vi "PCO_Grab_Save.vi"(7 "# of frames":u16, 8 "entrée d'erreur (pas d'erreur)":errorcluster, 9 "Message Data":variant, 10 "notifier out":refnum<notifier>, 11 "Camera en entrée":refnum<class "Camera.lvclass">) -> (0 "sortie d'erreur":errorcluster, 1 "meta_data_list":T1(array[cluster]), 2 "Raw data (U16)":u16[][][](array[numeric]), 3 "Camera en sortie":refnum<class "Camera.lvclass">)   [LabVIEW 2026]
uses:
  pco.labview/camera/Camera.lvclass
  Controls/PCO_Config.ctl
panel:
  out "recorded_image_count":u32
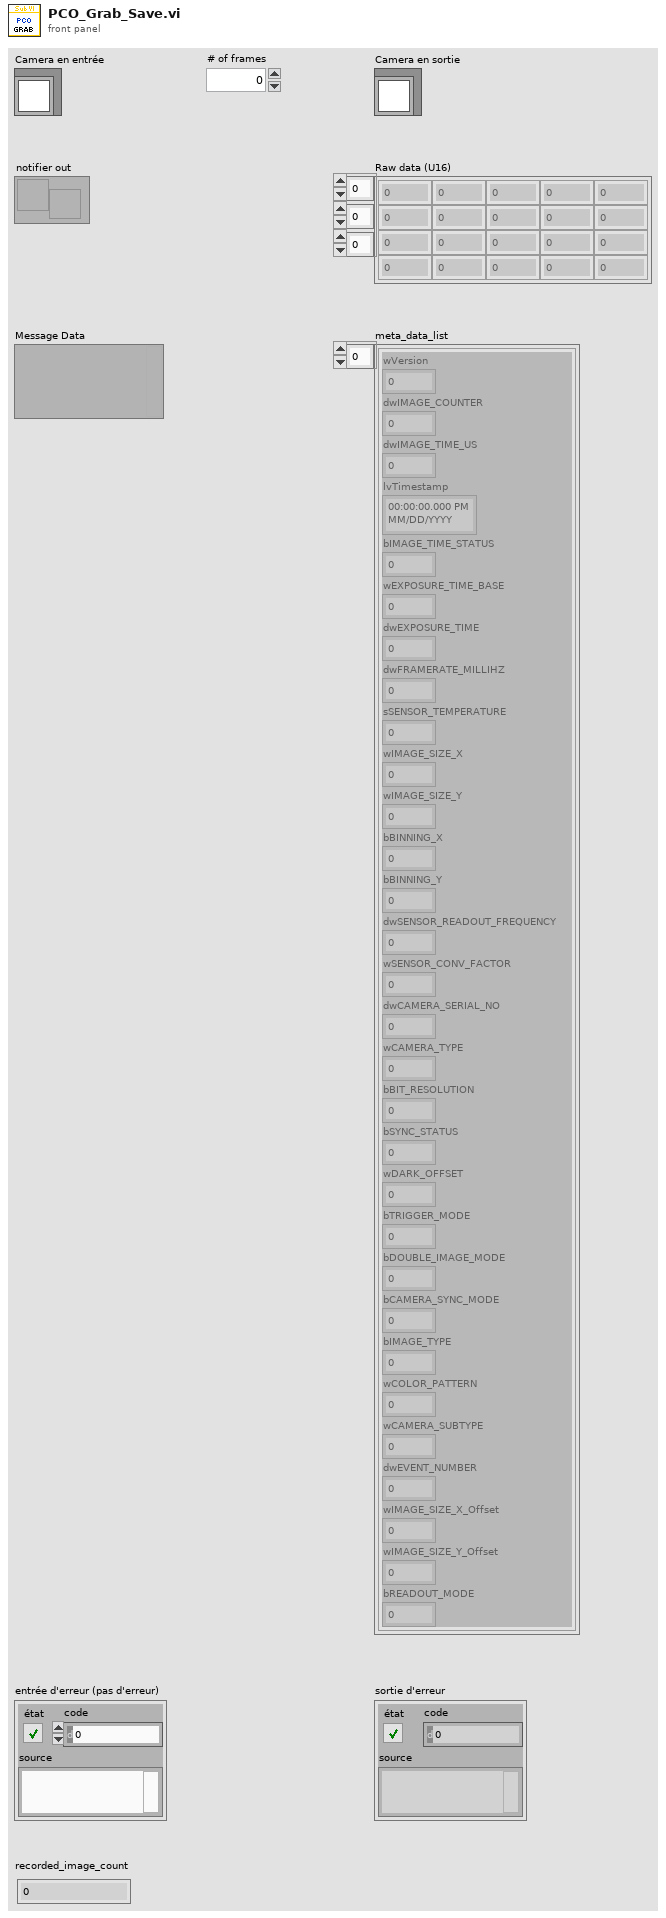
[diagram p1: front panel]
types:
  T1 = cluster{"wVersion":u16, "dwIMAGE_COUNTER":u32, "dwIMAGE_TIME_US":u32, "lvTimestamp":timestamp, "bIMAGE_TIME_STATUS":u8, "wEXPOSURE_TIME_BASE":u16, "dwEXPOSURE_TIME":u32, "dwFRAMERATE_MILLIHZ":u32, "sSENSOR_TEMPERATURE":i16, "wIMAGE_SIZE_X":u16, "wIMAGE_SIZE_Y":u16, "bBINNING_X":u8, "bBINNING_Y":u8, "dwSENSOR_READOUT_FREQUENCY":u32, "wSENSOR_CONV_FACTOR":u16, "dwCAMERA_SERIAL_NO":u32, "wCAMERA_TYPE":u16, "bBIT_RESOLUTION":u8, "bSYNC_STATUS":u8, "wDARK_OFFSET":u16, "bTRIGGER_MODE":u8, "bDOUBLE_IMAGE_MODE":u8, "bCAMERA_SYNC_MODE":u8, "bIMAGE_TYPE":u8, "wCOLOR_PATTERN":u16, "wCAMERA_SUBTYPE":u16, "dwEVENT_NUMBER":u32, "wIMAGE_SIZE_X_Offset":u16, "wIMAGE_SIZE_Y_Offset":u16, "bREADOUT_MODE":u8}[]
  T2 = enum16{"sequence", "sequence non blocking", "ring buffer", "fifo", "tif", "multitif", "pcoraw", "b16", "dicom", "multidicom", "camram_ring", "camram_segment"}
  T3 = enum16{"Undefined", "Mono8", "Mono16", "BGRA8", "RGBA8", "BGRA16", "RGBA16", "CompressedMono8"}
  T4 = typedef "PCO_Config.ctl" = cluster{"Exposure time (s)":dbl, "TriggerMode":u16, "ROI X0":u16, "ROI Y0":u16, "ROI X1":u16, "ROI Y1":u16, "Binning":u8}
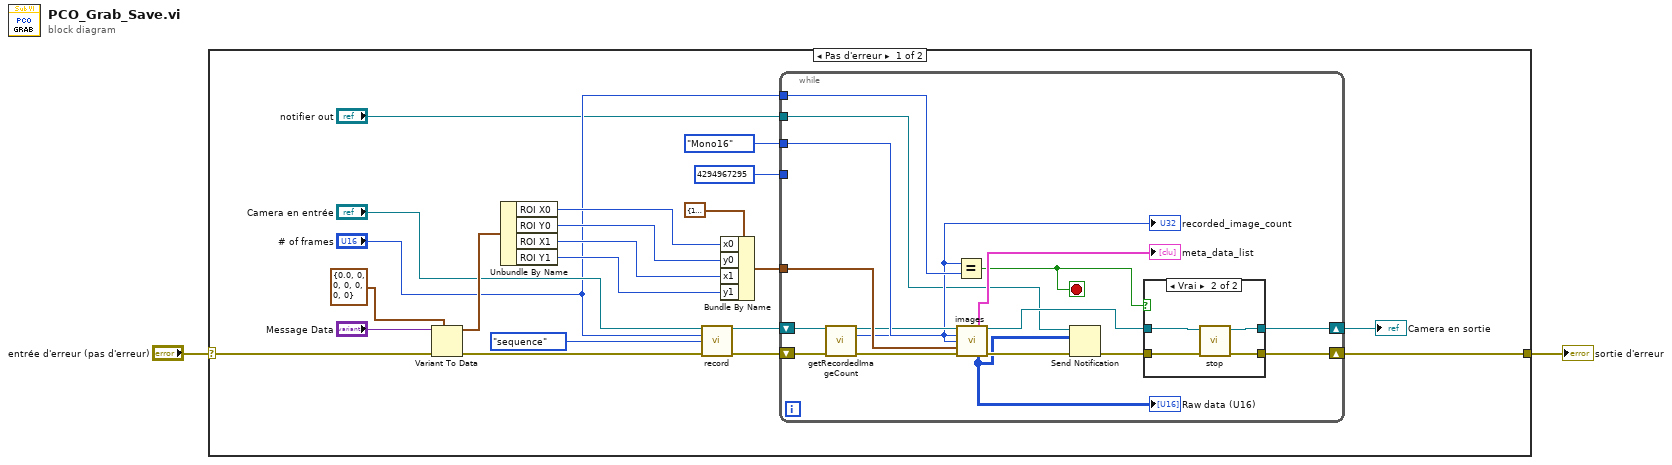
[diagram p0: block diagram]
diagram:
  n1 = case shown="Pas d'erreur" "entrée d'erreur (pas d'erreur)" {
    selector: "entrée d'erreur (pas d'erreur)" -> [w8 w47]
    tunnel: [w7 w47] -> w2
    frame No Error {
      n2 = Variant To Data(error in=w8, type=T4 {"Exposure time (s)"=0.0, "TriggerMode"=0, "ROI X0"=0, "ROI Y0"=0, "ROI X1"=0, "ROI Y1"=0, "Binning"=0} ("PCO_Config"), Variant="Message Data") -> (data=w17:T4, error out=w14:errorcluster)
      n3 = Unbundle By Name(w17) -> ("ROI X0"=w21:u16, "ROI Y0"=w20:u16, "ROI X1"=w19:u16, "ROI Y1"=w18:u16)
      n4 = call-dynamic "record.vi"("Camera in"="Camera en entrée", "num_images"="# of frames", "record_mode"=T2."sequence", "error in (no error)"=w14) -> ("Camera out"=w9:refnum<class "Camera.lvclass">, "error out"=w10:errorcluster)  [unwired: 10 in]
      n5 = Bundle By Name(cluster=cluster{"x0":u64, "y0":u64, "x1":u64, "y1":u64} {"x0"=18446744073709551615, "y0"=18446744073709551615, "x1"=18446744073709551615, "y1"=18446744073709551615} ("roi"), "x0"=w21, "y0"=w20, "x1"=w19, "y1"=w18) -> (w22:cluster{"x0":u64, "y0":u64, "x1":u64, "y1":u64})
      n6 = while {
        tunnel: T3."Mono16" ("data_format") -> [w40]
        tunnel: w22 -> [w39]
        tunnel: u32 4294967295 ("dwImgIdx") -> [_]
        shift-right: [w33] -> w7
        shift-left: w10 -> [w36]
        shift-right: [w30] -> w11
        shift-left: w9 -> [w35]
        tunnel: "# of frames" -> [w32]
        tunnel: "notifier out" -> [w26]
        stop <- w29 stop-if-true
        n7 = call-dynamic "getRecordedImageCount.vi"("Camera in"=w35, "error in (no error)"=w36) -> ("Camera out"=w37:refnum<class "Camera.lvclass">, "recorded_image_count"=w28:u32, "error out"=w38:errorcluster)  [unwired: 11 in]
        "recorded_image_count" <- w28
        n8 = Equal?(x=w28, y=w32) -> (x = y?=w29:bool)
        n9 = call-dynamic "images.vi"("Camera in"=w37, "data_format"=w40, "image_count"=w28, "crop"=w39, "error in (no error)"=w38) -> ("meta_data_list"=→"meta_data_list":T1, "Camera out"=w31:refnum<class "Camera.lvclass">, "raw_image_list (U16)"=w24:u16[][][], "error out"=w27:errorcluster)  [unwired: 2 in, 5 out]
        "Raw data (U16)" <- w24
        n10 = Send Notification(notification=w24, notifier=w26, error in (no error)=w27) -> (error out=w25:errorcluster)  [unwired: 1 out]
        n11 = case shown="Vrai" w29 {
          tunnel: w25 -> [w42 w46]
          tunnel: [w42 w45] -> w33
          tunnel: w31 -> [w41 w44]
          tunnel: [w41 w43] -> w30
          frame False {
          }
          frame True {
            n12 = call-dynamic "stop.vi"("error in (no error)"=w46, "Camera in"=w44) -> ("error out"=w45:errorcluster, "Camera out"=w43:refnum<class "Camera.lvclass">)  [unwired: 8 in]
          }
        }
      }
      "Camera en sortie" <- w11
    }
    frame Error {
    }
  }
  "sortie d'erreur" <- w2
